vi "Read Host Key Data.vi"(8 "error in (no error)":errorcluster, 11 "host key":T1) -> (0 "error out":errorcluster, 2 "host key data":T2)   [LabVIEW 2013, in "libssh2.lvlib"]
doc: "Read the data of a host key."
uses:
  libssh2.lvlib
  libssh2_knownhost.ctl
  Host Key Refnum.ctl
  Not A Host Key.vi
  <vilib>/Utility/error.llb/Error Cluster From Error Code.vi
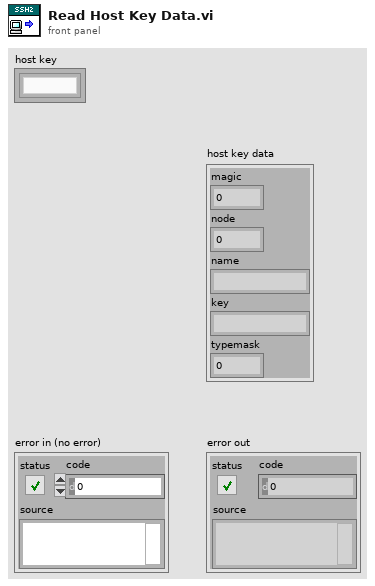
[diagram p1: front panel]
types:
  T1 = typedef "libssh2.lvlib/Host Key Refnum.ctl" = refnum<k1>
  T2 = typedef "libssh2.lvlib/libssh2_knownhost.ctl" = cluster{"magic":u32, "node":u64, "name":string, "key":string, "typemask":i32}
  T3 = cluster{"magic":u32, "node":u64, "name":u64, "key":u64, "typemask":i32}
  T4 = cluster{"magic":u32, "node":u32, "name":u32, "key":u32, "typemask":i32}
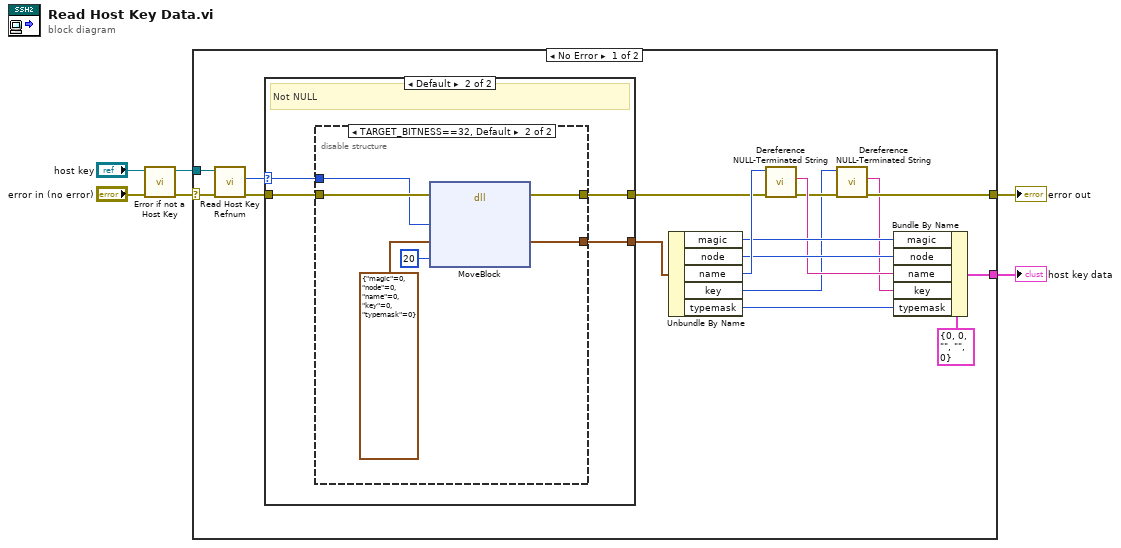
[diagram p0: block diagram]
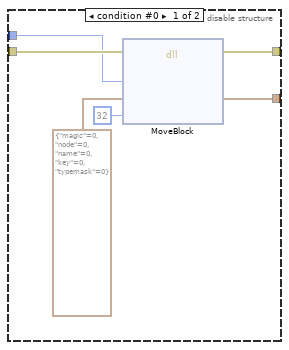
[diagram p3: hidden frame]
diagram:
  n1 = call "Error if not a Host Key.vi"("error in (no error)"="error in (no error)", "host key"="host key") -> ("error out"=w3:errorcluster, "host key out"=w1:T1)  [unwired: 8 in]
  n2 = case shown="No Error" w3 {
    selector: w3 -> [w13 w41]
    tunnel: [w23 _] -> w6
    tunnel: w1 -> [w20 _]
    tunnel: [w9 w41] -> w5
    frame No Error {
      n3 = call "Read Host Key Refnum.vi"("error in (no error)"=w13, "host key"=w20) -> ("error out"=w21:errorcluster, "libssh2_knownhost*"=w11:u64)  [unwired: 8 in]
      n4 = case shown="Default" w11 {
        selector: w11 -> [_ w25]
        tunnel: w21 -> [w24 w28]
        tunnel: [_ w27] -> w19
        tunnel: [w24 w26] -> w12
        frame 0 {
          # "NULL"
        }
        frame Default {
          # "Not NULL"
          n5 = disable-structure shown="TARGET_BITNESS==32, Default" {
            disable-tunnel: w28 -> [w34 w40]
            disable-tunnel: [w32 w38] -> w27
            disable-tunnel: [w31 w37] -> w26
            disable-tunnel: w25 -> [w30 w36]
            frame condition #0 {
              n6 = dll-call lib="LabVIEW" fn="MoveBlock"(error in=w34, "ps"=w30, T3 {"magic"=0, "node"=0, "name"=0, "key"=0, "typemask"=0}, "size"=i64 32) -> (error out=w31:errorcluster, w32:T3)  [unwired: 5 in, 1 out]
            }
            frame condition #1 (active) {
              n7 = dll-call lib="LabVIEW" fn="MoveBlock"(error in=w40, "ps"=w36, T4 {"magic"=0, "node"=0, "name"=0, "key"=0, "typemask"=0}, "size"=i64 20) -> (error out=w37:errorcluster, w38:T4)  [unwired: 5 in, 1 out]
            }
          }
        }
      }
      n8 = Unbundle By Name(w19) -> ("magic"=w17:u32, "node"=w16:u32, "name"=w18:u32, "key"=w8:u32, "typemask"=w14:i32)
      n9 = call "Dereference NULL-Terminated String.vi"("error in (no error)"=w12, "char*"=w18) -> ("error out"=w10:errorcluster, "string"=w15:string)  [unwired: 8 in]
      n10 = call "Dereference NULL-Terminated String.vi"("error in (no error)"=w10, "char*"=w8) -> ("error out"=w9:errorcluster, "string"=w7:string)  [unwired: 8 in]
      n11 = Bundle By Name(cluster=T2 {"magic"=0, "node"=0, "name"="", "key"="", "typemask"=0} ("libssh2_knownhost"), "magic"=w17, "node"=w16, "name"=w15, "key"=w7, "typemask"=w14) -> (w23:T2)
    }
    frame Error {
    }
  }
  "host key data" <- w6
  "error out" <- w5
